vi "clusters.vi"() -> ()   [LabVIEW 2017]
panel:
  out "array of clusters":T1(array[cluster])
  in  "stop":bool
  out "Cluster 3":T2
  in  "String":string
  in  "Boolean":bool
  in  "Numeric":dbl
  out "Cluster 2":T2
  in  "Cluster":T3
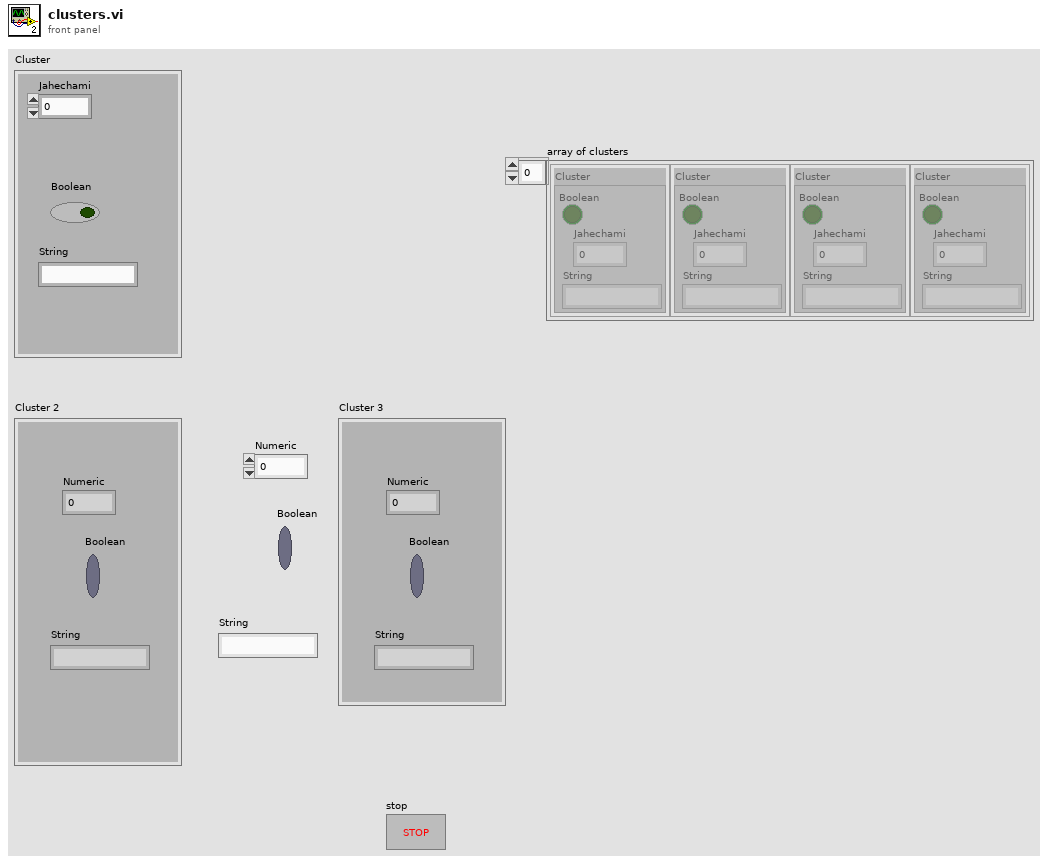
[diagram p1: front panel]
types:
  T1 = cluster{"Cluster":cluster{"Boolean":bool, "Jahechami":dbl, "String":string}}[]
  T2 = cluster{"Boolean":bool, "Numeric":dbl, "String":string}
  T3 = cluster{"Boolean":bool, "Jahechami":dbl, "String":string}
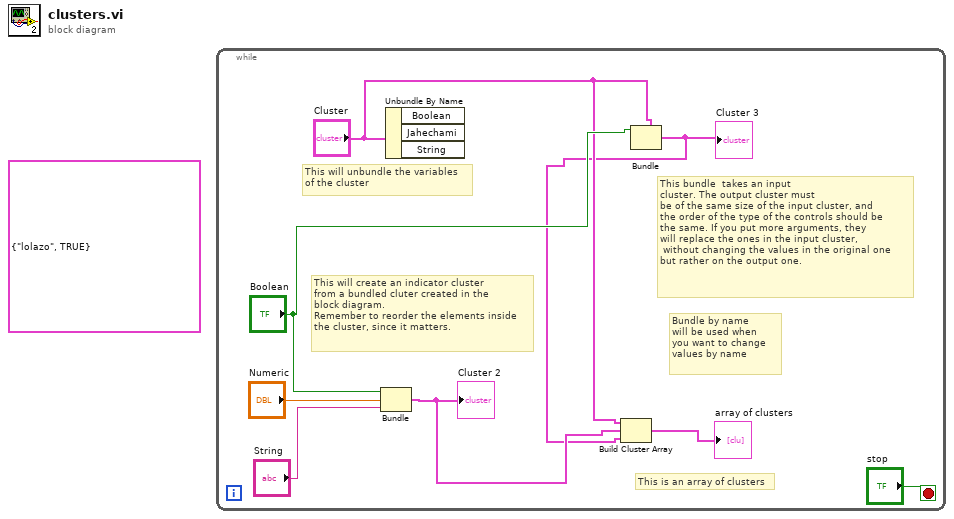
[diagram p0: block diagram]
diagram:
  (unwired) cluster{string, bool} {"lolazo", TRUE}
  n1 = while {
    stop <- "stop" stop-if-true
    # "This is an array of clusters"
    # "Bundle by name \nwill be used when \nyou want to change \nvalues by name"
    # "This bundle  takes an input\ncluster. The output cluster must\nbe of the same size of the input cluster, and\nthe order of the type of the controls should be\nthe same. If you put more arguments, they\nwill replace the ones in the input cluster,\n without changing the values in the original one\nbut rather on the output one."
    # "This will create an indicator cluster\nfrom a bundled cluter created in the \nblock diagram.\nRemember to reorder the elements inside\nthe cluster, since it matters."
    # "This will unbundle the variables\nof the cluster"
    n2 = Bundle("Boolean"="Boolean", "Numeric"="Numeric", "String"="String") -> (w3:T2)  [unwired: 1 in]
    "Cluster 2" <- w3
    n3 = Unbundle By Name("Cluster") -> ()  [unwired: 3 out]
    n4 = Bundle(cluster="Cluster", "Boolean"="Boolean") -> (w1:T3)  [unwired: 2 in]
    "Cluster 3" <- w1
    n5 = Build Cluster Array("Cluster", w3, w1) -> (→"array of clusters":T1)
  }
